vi "RT_Number_Of_Connections.vi"(8 "Error In":errorcluster, 11 "Counter_FGV_States":T1) -> (0 "Error Out":errorcluster, 3 "Number of connections":i32)   [LabVIEW 2018]
uses:
  RT_Counter_FGV_States.ctl
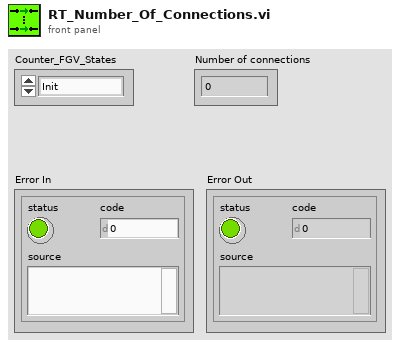
[diagram p1: front panel]
types:
  T1 = typedef "RT_Counter_FGV_States.ctl" = enum16{"Init", "Increase", "Decrease", "Get"}
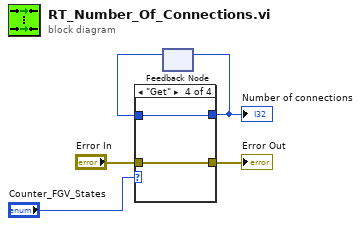
[diagram p0: block diagram]
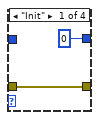
[diagram p2: hidden frame]
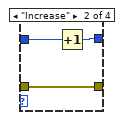
[diagram p3: hidden frame]
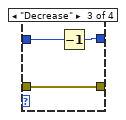
[diagram p4: hidden frame]
diagram:
  n1 = feedback #1() -> (w2:i32)  [unwired: 1 in]
  n2 = case shown="\"Get\"" "Counter_FGV_States" {
    tunnel: [w6 w10 w11 w14] -> w5
    tunnel: "Error In" -> [w6 w10 w11 w14]
    tunnel: [0 w8 w12 w15] -> w1
    tunnel: w2 -> [_ w9 w13 w15]
    frame "Init" {
    }
    frame "Increase" {
      n3 = Increment(x=w9) -> (x+1=w8:i32)
    }
    frame "Decrease" {
      n4 = Decrement(x=w13) -> (x-1=w12:i32)
    }
    frame "Get" {
    }
  }
  "Error Out" <- w5
  "Number of connections" <- w1
  n5 = feedback-in #1(w1) -> ()
